vi "get_status.vi"(8 "error in (no error)":errorcluster, 11 "Keithley2002 in":refnum<class "Keithley2002.lvclass">) -> (0 "error out":errorcluster, 2 "status":cluster{"status":bool, "source":string}={"status"=TRUE, "source"=""}, 3 "Keithley2002 out":refnum<class "Keithley2002.lvclass">)   [LabVIEW 2019, in "Keithley2002.lvclass"]
uses:
  Keithley2002.lvclass
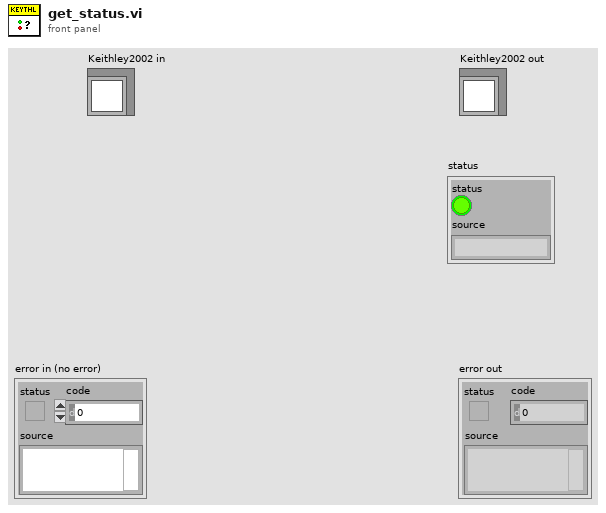
[diagram p1: front panel]
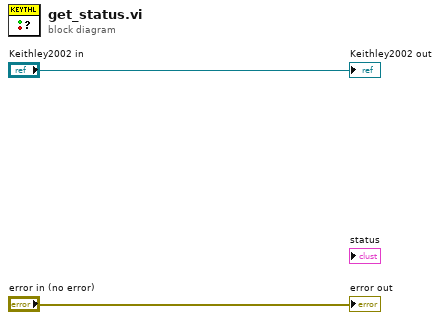
[diagram p0: block diagram]
diagram:
  "error out" <- "error in (no error)"
  "Keithley2002 out" <- "Keithley2002 in"
